vi "Array 2 Actuator Controls.vi"(10 "Array":dbl[](array[numeric])) -> (2 "Actuator Controls":T1 {"Actuator Z2" min=-10.0 max=10.0 step=0.1 scale=-10.0..10.0; "Actuator Z3" min=-10.0 max=10.0 step=0.1 scale=-10.0..10.0; "Actuator X2" min=-10.0 max=10.0 step=0.1 scale=-10.0..10.0; "Actuator Y1" min=-10.0 max=10.0 step=0.1 scale=-10.0..10.0; "Actuator Z1" min=-10.0 max=10.0 step=0.1 scale=-10.0..10.0; "Actuator X1" min=-10.0 max=10.0 step=0.1 scale=-10.0..10.0})   [LabVIEW 2009]
uses:
  Actuator Controls.ctl
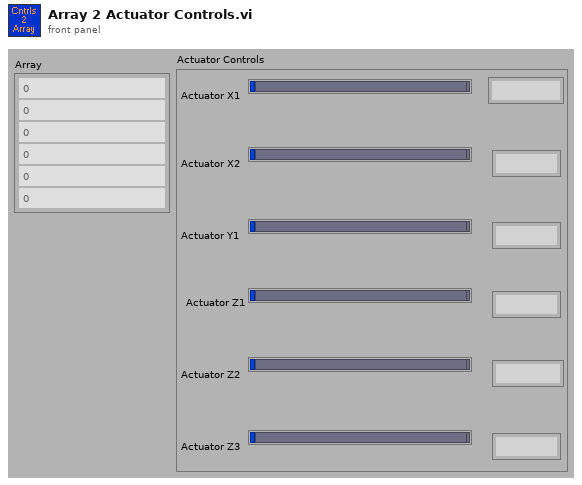
[diagram p1: front panel]
types:
  T1 = typedef "Actuator Controls.ctl" = cluster{"Actuator X1":dbl, "Actuator X2":dbl, "Actuator Y1":dbl, "Actuator Z1":dbl, "Actuator Z2":dbl, "Actuator Z3":dbl}
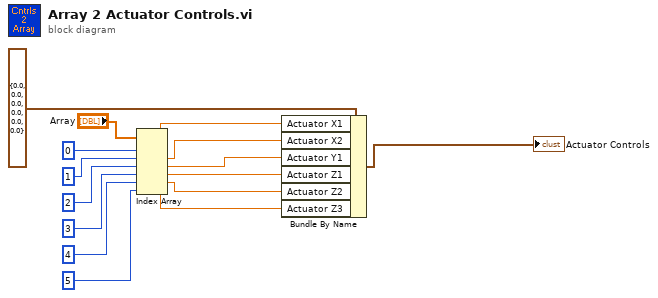
[diagram p0: block diagram]
diagram:
  n1 = Index Array(array="Array", index #1=0 ("index"), index #2=1 ("index"), index #3=2 ("index"), index #4=3 ("index"), index #5=4 ("index"), index #6=5 ("index")) -> (element #1=w7:dbl, element #2=w6:dbl, element #3=w5:dbl, element #4=w4:dbl, element #5=w3:dbl, element #6=w2:dbl)
  n2 = Bundle By Name(cluster=T1 {"Actuator X1"=0.0, "Actuator X2"=0.0, "Actuator Y1"=0.0, "Actuator Z1"=0.0, "Actuator Z2"=0.0, "Actuator Z3"=0.0} ("Actuator Controls"), "Actuator X1"=w7, "Actuator X2"=w6, "Actuator Y1"=w5, "Actuator Z1"=w4, "Actuator Z2"=w3, "Actuator Z3"=w2) -> (→"Actuator Controls":T1)
